vi "setHistogram.vi"(8 "Auto. In":bool=TRUE, 9 "max counts":dbl, 10 "bins":dbl, 11 "WaveformGraph in":refnum<vi>) -> (0 "Auto. Out":bool=TRUE)   [LabVIEW 2022 SP3]
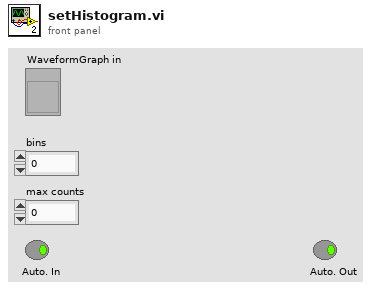
[diagram p1: front panel]
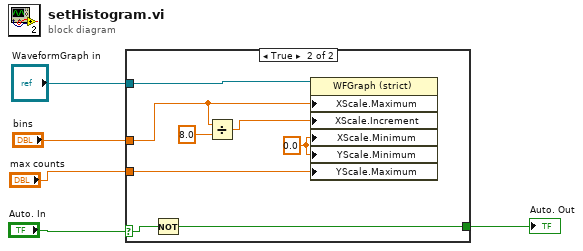
[diagram p0: block diagram]
diagram:
  n1 = case shown="True" "Auto. In" {
    selector: "Auto. In" -> [w6 w13]
    tunnel: "WaveformGraph in" -> [_ w14]
    tunnel: [w6 w12] -> w3
    tunnel: "bins" -> [_ w8]
    tunnel: "max counts" -> [_ w10]
    frame False {
    }
    frame True {
      w11 = 0.0 ("Y Scale.Range:Minimum")
      n2 = Not(x=w13) -> (.not. x?=w12:bool)
      n3 = Divide(x=w8, y=8.0) -> (x/y=w9:dbl)
      n4 = property on="Property Node" class="WFGraph (strict)"(reference=w14, "XScale.Maximum"=w8, "XScale.Increment"=w9, "XScale.Minimum"=w11, "YScale.Minimum"=w11, "YScale.Maximum"=w10) -> ()  [unwired: 1 in, 2 out]
    }
  }
  "Auto. Out" <- w3
